vi "Cal ColNum(SubVI).vi"(4 "StartOfImage":bool, 6 "Ready For Input":bool, 8 "Width":i16, 9 "EOL":bool, 10 "DV":bool, 11 "curColNum":i16) -> (3 "nextColNum":i16)   [LabVIEW 2016]
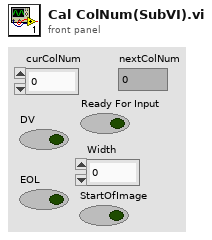
[diagram p1: front panel]
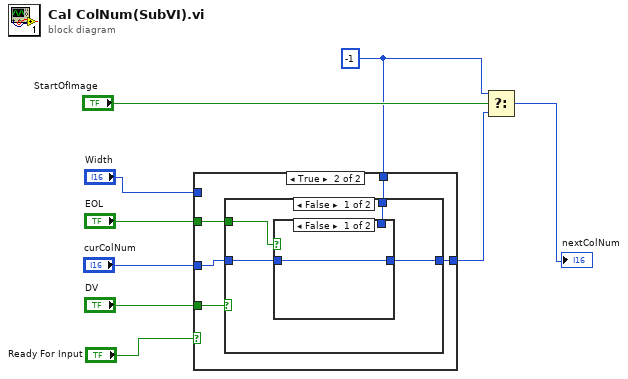
[diagram p0: block diagram]
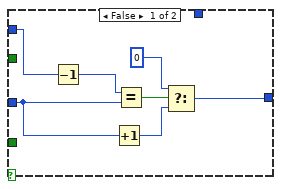
[diagram p2: hidden frame]
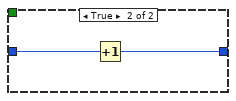
[diagram p4: hidden frame]
diagram:
  w1 = i16 -1 ("t")
  n1 = case shown="True" "Ready For Input" {
    tunnel: [w12 w21] -> w3
    tunnel: "DV" -> [_ w20]
    tunnel: "curColNum" -> [w14 w19]
    tunnel: "EOL" -> [_ w18]
    tunnel: "Width" -> [w11 _]
    tunnel: w1 -> [_ w17]
    frame False {
      n2 = Decrement(x=w11) -> (x-1=w10:i16)
      n3 = Increment(x=w14) -> (x+1=w15:i16)
      n4 = Equal?(x=w10, y=w14) -> (x = y?=w16:bool)
      n5 = Select(t=i16 0, s=w16, f=w15) -> (s? t:f=w12:i16)
    }
    frame True {
      n6 = case shown="False" w20 {
        tunnel: w18 -> [w25 _]
        tunnel: [w24 w29] -> w21
        tunnel: w19 -> [w23 w28]
        tunnel: w17 -> [w22 _]
        frame False {
          n7 = case shown="False" w25 {
            tunnel: [w26 w27] -> w24
            tunnel: w23 -> [w26 _]
            tunnel: w22 -> [_ w27]
            frame False {
            }
            frame True {
            }
          }
        }
        frame True {
          n8 = Increment(x=w28) -> (x+1=w29:i16)
        }
      }
    }
  }
  n9 = Select(t=w1, s="StartOfImage", f=w3) -> (s? t:f=→"nextColNum":i16)
